vi "hcE.vi"(10 "partition":i32[](array[numeric]), 11 "data":dbl[][](array[numeric])) -> (0 "modelName":string, 1 "dim":i32, 2 "initialPartition":i32[](array[numeric]), 3 "hcPair":dbl[][](array[numeric]))   [LabVIEW 2014]
panel:
  out "data (1D)":dbl[](array[numeric])
  out "Error Message":string
  out "Id":dbl
  out "m":i32
  out "II":dbl
  out "I":i32
  out "oneD":bool
  out "n":i32
  in  "minclus":i32=1
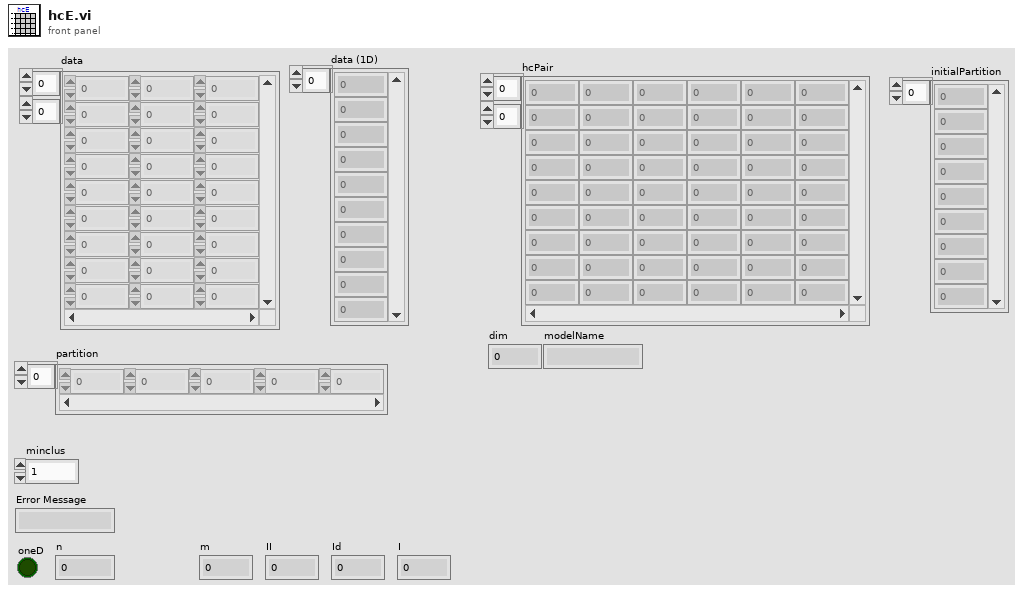
[diagram p1: front panel]
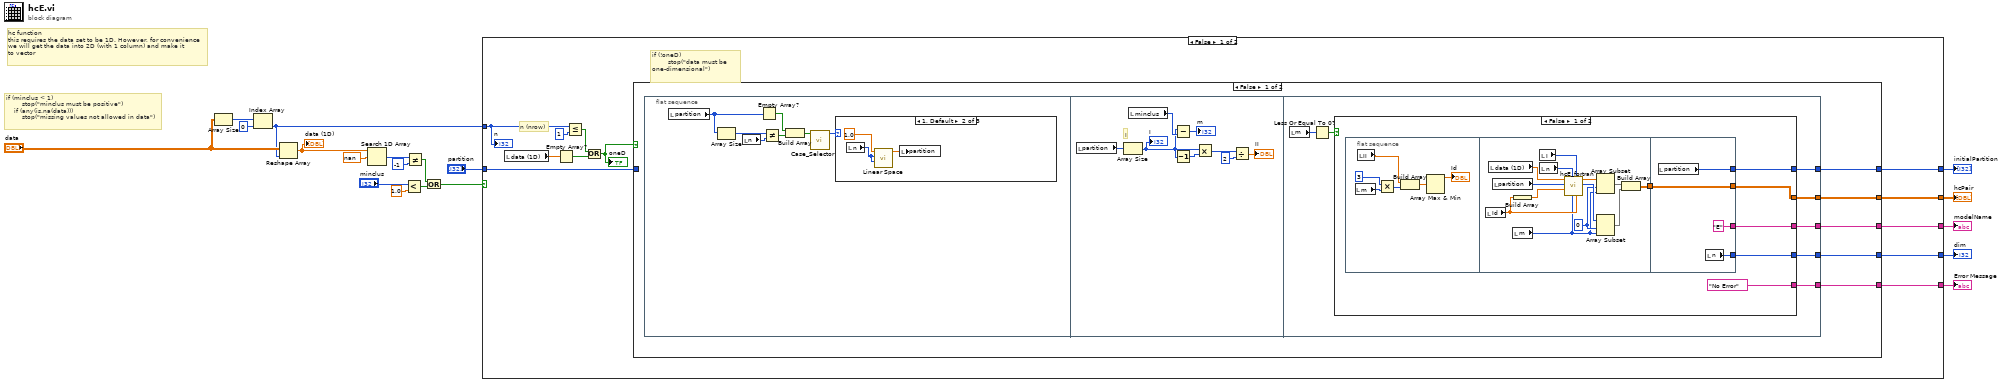
[diagram p0: block diagram]
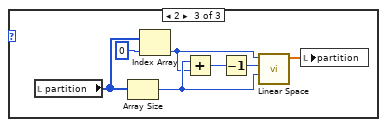
[diagram p3: hidden frame]
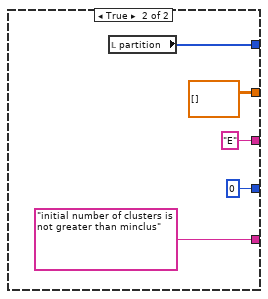
[diagram p4: hidden frame]
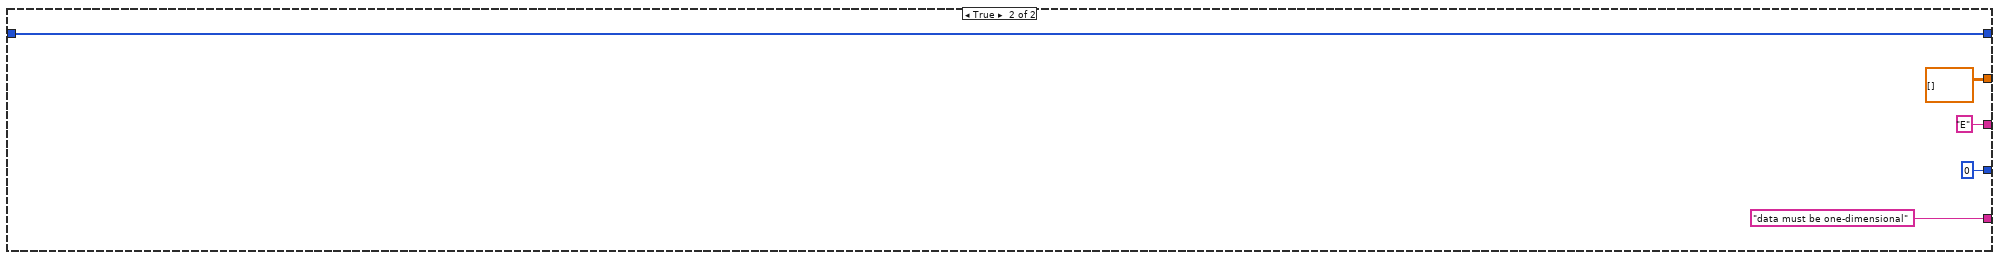
[diagram p5: hidden frame]
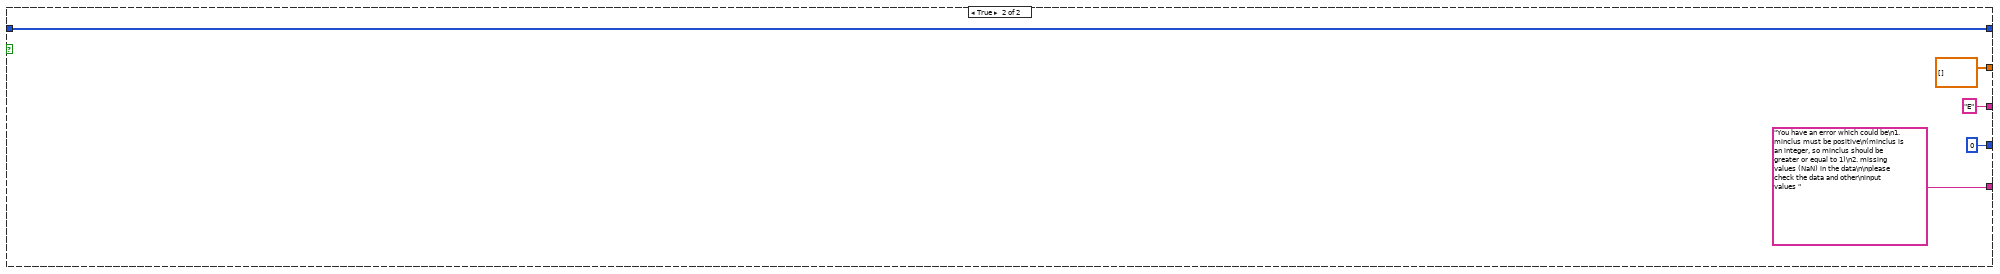
[diagram p6: hidden frame]
diagram:
  # "if (minclus < 1) \n        stop(\"minclus must be positive\")\n    if (any(is.na(data))) \n        stop(\"missing values not allowed in data\")"
  # "hc function\nthis requires the data set to be 1D. However, for convenience\nwe will get the data into 2D (with 1 column) and make it\nto vector"
  n1 = Array Size(array="data") -> (size(s)=w7:i32[])
  n2 = Index Array(array=w7, index=0) -> (element=w5:i32)
  n3 = Reshape Array("data", w5) -> (w17:dbl[])
  "data (1D)" <- w17
  n4 = Search 1D Array(1D array=w17, element=nan) -> (index of element=w15:i32)  [unwired: 1 in]
  n5 = Less?(x="minclus", y=1.0) -> (x < y?=w12:bool)
  n6 = Not Equal?(x=w15, y=-1) -> (x != y?=w13:bool)
  n7 = Or(x=w13, y=w12) -> (x .or. y?=w11:bool)
  n8 = case shown="False" w11 {
    tunnel: [w31 dbl[][] [] ("data")] -> w9
    tunnel: [w30 "You have an error which could be\n1. minclus must be positive\n(minclus is an integer, so minclus should be greater or equal to 1)\n2. missing values (NaN) in the data\n\nplease check the data and other\ninput values "] -> w8
    tunnel: w5 -> [w27 _]
    tunnel: [w23 w108] -> w4
    tunnel: [w22 0 ("n")] -> w3
    tunnel: [w21 "E"] -> w2
    tunnel: "partition" -> [w20 w108]
    frame False {
      # "n (nrow)"
      # "if (!oneD) \n        stop(\"data must be one-dimensional\")"
      n9 = local read "data (1D)"() -> (w25:dbl[])
      n10 = Empty Array?(array=w25) -> (empty?=w26:bool)
      n11 = Less Or Equal?(x=w27, y=1) -> (x <= y?=w29:bool)
      n12 = Or(x=w29, y=w26) -> (x .or. y?=w24:bool)
      "oneD" <- w24
      n13 = case shown="False" w24 {
        tunnel: [w36 dbl[][] [] ("data")] -> w31
        tunnel: [w35 "data must be one-dimensional"] -> w30
        tunnel: [w34 w103] -> w23
        tunnel: [w33 0 ("n")] -> w22
        tunnel: [w32 "E"] -> w21
        tunnel: w20 -> [_ w103]
        frame False {
          n14 = flat-sequence {
            tunnel: [w66] -> w36
            tunnel: [w65] -> w35
            tunnel: [w64] -> w34
            tunnel: [w63] -> w33
            tunnel: [w62] -> w32
            frame #0 {
              n15 = local read "partition"() -> (w43:i32[])
              n16 = Array Size(array=w43) -> (size(s)=w41:i32)
              n17 = local read "n"() -> (w42:i32)
              n18 = Empty Array?(array=w43) -> (empty?=w40:bool)
              n19 = Not Equal?(x=w41, y=w42) -> (x != y?=w39:bool)
              n20 = Build Array(w40, w39) -> (w38:bool[])
              n21 = call "Case_Selector.vi"("Array"=w38) -> ("Case Numer"=w37:i32)  [unwired: 10 in]
              n22 = case shown="1, Default" w37 {
                frame 0 {
                }
                frame 1, Default {
                  n23 = local read "n"() -> (w44:i32)
                  n24 = call "Linear Space.vi"("Number of Samples"=w44, "Maximum"=w44, "Minimum"=1.0) -> ("Array"=w46:dbl[])  [unwired: 3 in, 1 out]
                  n25 = local write "partition"(w46) -> ()
                }
                frame 2 {
                  n26 = local read "partition"() -> (w51:i32[])
                  n27 = Array Size(array=w51) -> (size(s)=w50:i32)
                  n28 = Index Array(array=w51, index=0) -> (element=w49:i32)
                  n29 = Add(x=w50, y=w49) -> (x+y=w48:i32)
                  n30 = Decrement(x=w48) -> (x-1=w47:i32)
                  n31 = call "Linear Space.vi"("Number of Samples"=w50, "Maximum"=w47, "Minimum"=w49) -> ("Array"=w53:dbl[])  [unwired: 3 in, 1 out]
                  n32 = local write "partition"(w53) -> ()
                }
              }
            }
            frame #1 {
              # "I"
              n33 = local read "partition"() -> (w61:i32[])
              n34 = Array Size(array=w61) -> (size(s)=w57:i32)
              "I" <- w57
              n35 = local read "minclus"() -> (w60:i32)
              n36 = Subtract(x=w57, y=w60) -> (x-y=→"m":i32)
              n37 = Decrement(x=w57) -> (x-1=w58:i32)
              n38 = Multiply(x=w57, y=w58) -> (x*y=w56:i32)
              n39 = Divide(x=w56, y=2) -> (x/y=→"II":dbl)
            }
            frame #2 {
              n40 = local read "m"() -> (w68:i32)
              n41 = Less Or Equal To 0?(x=w68) -> (x <= 0?=w67:bool)
              n42 = case shown="False" w67 {
                tunnel: [w73 dbl[][] [] ("data")] -> w66
                tunnel: ["No Error" "initial number of clusters is not greater than minclus"] -> w65
                tunnel: [w71 w98] -> w64
                tunnel: [w70 0 ("n")] -> w63
                tunnel: [w69 "E"] -> w62
                frame False {
                  n43 = flat-sequence {
                    tunnel: [w81] -> w72
                    tunnel: [w97] -> w73
                    tunnel: w72 -> [w97]
                    tunnel: [w96] -> w71
                    tunnel: [w95] -> w70
                    tunnel: ["E"] -> w69
                    frame #0 {
                      n44 = local read "m"() -> (w80:i32)
                      n45 = local read "II"() -> (w75:dbl)
                      n46 = Multiply(x=3, y=w80) -> (x*y=w76:i32)
                      n47 = Build Array(w75, w76) -> (w78:dbl[])
                      n48 = Array Max & Min(array=w78) -> (max value=→"Id":dbl)  [unwired: 3 out]
                    }
                    frame #1 {
                      w85 = 0
                      n49 = local read "Id"() -> (w89:dbl)
                      n50 = local read "data (1D)"() -> (w93:dbl[])
                      n51 = local read "partition"() -> (w91:i32[])
                      n52 = local read "m"() -> (w84:i32)
                      n53 = Build Array(w89) -> (w88:dbl[])
                      n54 = local read "I"() -> (w90:i32)
                      n55 = local read "n"() -> (w92:i32)
                      n56 = call "hcE_fortran.vi"("nd"=w89, "ng"=w90, "ns"=w84, "n"=w92, "d"=w88, "ic"=w91, "x (data)"=w93) -> ("ic (out)"=w86:i32[], "x (data out)"=w87:dbl[])  [unwired: 2 in, 1 out]
                      n57 = Array Subset(array=w87, index=w85, length=w84) -> (w83:dbl[])
                      n58 = Array Subset(array=w86, index=w85, length=w84) -> (w82:i32[])
                      n59 = Build Array(w83, w82) -> (w81:dbl[][])
                    }
                    frame #2 {
                      n60 = local read "partition"() -> (w96:i32[])
                      n61 = local read "n"() -> (w95:i32)
                    }
                  }
                }
                frame True {
                  n62 = local read "partition"() -> (w98:i32[])
                }
              }
            }
          }
        }
        frame True {
        }
      }
      "n" <- w27
    }
    frame True {
    }
  }
  "hcPair" <- w9
  "Error Message" <- w8
  "initialPartition" <- w4
  "dim" <- w3
  "modelName" <- w2
